vi "Open.vi"(8 "error in (no error)":errorcluster, 11 "File in":refnum<class "File.lvclass">) -> (0 "error out":errorcluster, 3 "File out":refnum<class "File.lvclass">)   [LabVIEW 2019, in "File.lvclass"]
uses:
  File.lvclass
  File.lvclass/File.ctl
  Read Data File  Path.vi
  Read Is open.vi
  Read tdms stream.vi
  Write tdms stream.vi
  Write Is open.vi
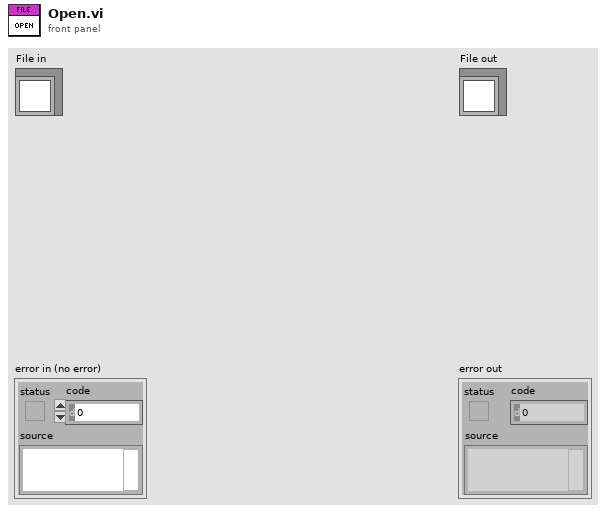
[diagram p1: front panel]
types:
  T1 = enum16{"open", "open or create", "create or replace", "create", "open (read-only)"}
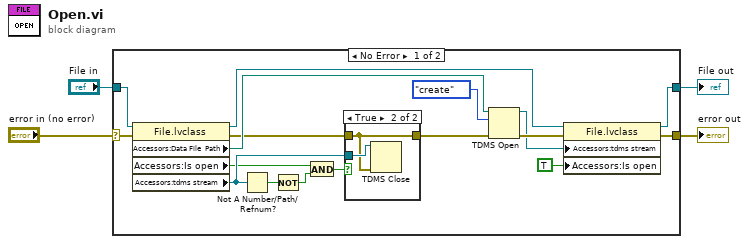
[diagram p0: block diagram]
diagram:
  n1 = case shown="No Error" "error in (no error)" {
    selector: "error in (no error)" -> [w21 w26]
    tunnel: [w11 w26] -> w3
    tunnel: [w9 w25] -> w1
    tunnel: "File in" -> [w20 w25]
    frame No Error {
      n2 = property class="File.lvclass"(reference=w20, error in=w21) -> (reference out=w10:refnum<class "File.lvclass">, error out=w6:errorcluster, "Accessors:Data File  Path"=w14:path, "Accessors:Is open"=w15:bool, "Accessors:tdms stream"=w17:refnum<k34>)
      n3 = Not A Number/Path/Refnum?(number/path/refnum=w17) -> (NaN/Path/Refnum?=w18:bool)
      n4 = Not(x=w18) -> (.not. x?=w19:bool)
      n5 = And(x=w15, y=w19) -> (x .and. y?=w16:bool)
      n6 = case shown="True" w16 {
        tunnel: w6 -> [w22 w23]
        tunnel: w17 -> [_ w24]
        tunnel: [w22 w23] -> w5
        frame False {
        }
        frame True {
          n7 = TDMS Close(8:w23, 11:w24) -> ()  [unwired: 2 out]
        }
      }
      n8 = TDMS Open(8:w5, 10:T1."create" ("operation (0:open)"), 11:w14) -> (0:w12:errorcluster, 3:w8:refnum<k34>)  [unwired: 4 in]
      n9 = property class="File.lvclass"(reference=w10, error in=w12, "Accessors:tdms stream"=w8, "Accessors:Is open"=TRUE ("Is open")) -> (reference out=w9:refnum<class "File.lvclass">, error out=w11:errorcluster)
    }
    frame Error {
    }
  }
  "error out" <- w3
  "File out" <- w1
